vi "getInheritanceChain.vi"(8 "error in (no error)":errorcluster, 11 "GraphNode in":refnum<class "GraphNode.lvclass">) -> (0 "error out":errorcluster, 2 "Inheritance Chain":string[](array[string]), 3 "GraphNode out":refnum<class "GraphNode.lvclass">)   [LabVIEW 2009, in "GraphNode.lvclass"]
doc: "Returns the inheritance chain."
uses:
  GraphNode.lvclass
  Node/Node.lvclass
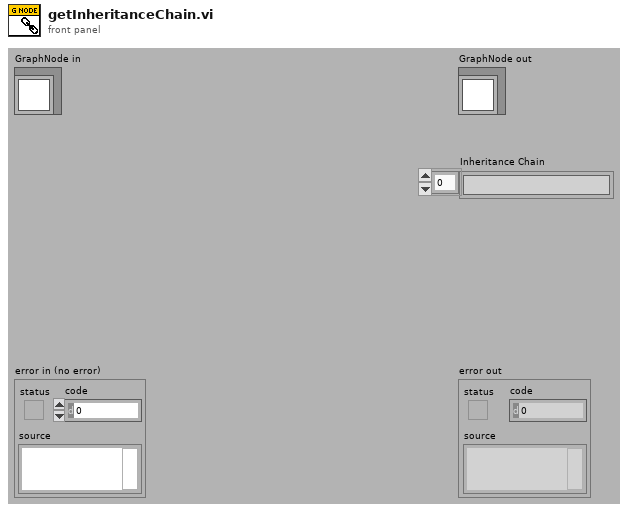
[diagram p1: front panel]
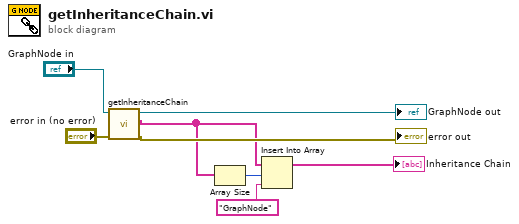
[diagram p0: block diagram]
diagram:
  n1 = call-parent "getInheritanceChain.vi"("error in (no error)"="error in (no error)", "Node in"="GraphNode in") -> ("error out"=→"error out":errorcluster, "Inheritance Chain"=w3:string[], "Node out"=→"GraphNode out":refnum<class "GraphNode.lvclass">)  [unwired: 7 in]
  n2 = Array Size(array=w3) -> (size(s)=w6:i32)
  n3 = Insert Into Array(array=w3, index=w6, new element="GraphNode") -> (→"Inheritance Chain":string[])
